vi "part-b.vi"(1 "Compunded":u16(ring) items=["yearly"=1, "half yearly"=2, "quarterly"=4, "monthly"=12, "bi-weekly"=26, "weekly"=52, "daily"=109], 2 "Annual Interest Rate(%)":dbl) -> (0 "Rate of Y1":dbl)   [LabVIEW 2021]
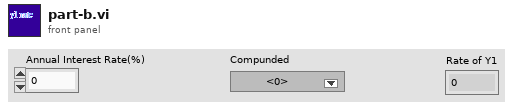
[diagram p1: front panel]
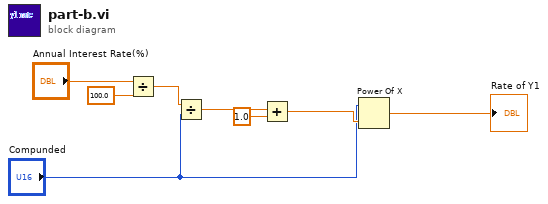
[diagram p0: block diagram]
diagram:
  n1 = Divide(x="Annual Interest Rate(%)", y=100.0) -> (x/y=w2:dbl)
  n2 = Divide(x=w2, y="Compunded") -> (x/y=w8:dbl)
  n3 = Add(x=w8, y=1.0) -> (x+y=w6:dbl)
  n4 = Power Of X(1:w6, 2:"Compunded") -> (0:→"Rate of Y1":dbl)
